vi "文本文件（格式化写入）.vi"   [LabVIEW 2017]
types:
  T1 = enum16{"open", "replace", "create", "open or create", "replace or create", "replace or create with confirmation"}
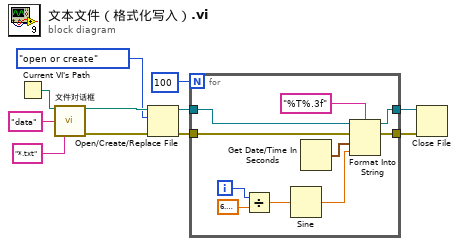
[diagram p0: block diagram]
diagram:
  n1 = Current VI's Path() -> (path=w9:path)
  n2 = call "文件对话框"("start path"=w9, "default name"="data", "pattern (all files)"="*.txt") -> ("selected path"=w8:path, "error out"=w7:errorcluster)  [unwired: 9 in, 2 out]
  n3 = Open/Create/Replace File(file path (use dialog)=w8, error in=w7, operation (0:open)=T1."open or create" ("操作(0:open)")) -> (refnum out=w4:refnum<file>, error out=w3:errorcluster)  [unwired: 3 in, 1 out]
  n4 = for {
    N: 100 -> [_]
    tunnel: w4 -> [w21]
    tunnel: w3 -> [w20]
    tunnel: [w13] -> w2
    tunnel: [w12] -> w1
    i -> [w15]
    n5 = Divide(x=w15, y=6.283185307179586) -> (x/y=w17:dbl)
    n6 = Sine(x=w17) -> (sin(x)=w14:dbl)
    n7 = Get Date/Time In Seconds() -> (seconds since 1Jan1904=w18:timestamp)
    n8 = Format Into String(format string="%T%.3f" ("格式字符串"), initial string=w21, error in=w20, w18, w14) -> (resulting string=w13:refnum<file>, error out=w12:errorcluster)
  }
  n9 = Close File(refnum=w2, error in=w1) -> ()  [unwired: 2 out]
